vi "timerfd_settime.vi"(8 "error in (no error)":errorcluster, 10 "new value":T1, 11 "fd in":i32) -> (0 "error out":errorcluster, 2 "old value":T1, 3 "fd out":i32)   [LabVIEW 2013, in "Linux RT IPC.C.lvlib"]
uses:
  Linux RT IPC.C.lvlib
  Controls/functions.ctl
  <vilib>/NI/NI Linux RT Errno/Linux Errno.lvlib
  <vilib>/NI/NI Linux RT Utilities/Linux RT Utilities.lvlib
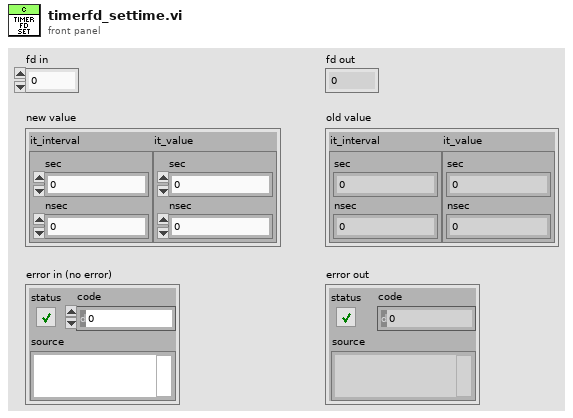
[diagram p1: front panel]
types:
  T1 = cluster{"it_interval":cluster{"sec":u64, "nsec":u64}, "it_value":cluster{"sec":u64, "nsec":u64}}
  T2 = cluster{"it_interval":cluster{"sec":u32, "nsec":u32}, "it_value":cluster{"sec":u32, "nsec":u32}}
  T3 = cluster{"timespec 64":cluster{"sec":u64, "nsec":u64}, "timespec 64":cluster{"sec":u64, "nsec":u64}}
  T4 = typedef "Linux RT IPC.C.lvlib/functions.ctl" = enum16{"unspecified", "close", "epoll_create", "epoll_ctl", "epoll_wait", "fstat", "ftruncate", "mkfifo", "mmap", "munmap", "open", "read", "shm_open", "shm_unlink", "timerfd_create", "timerfd_settime", "timerfd_gettime", "write", "unlink"}
  T5 = typedef "Linux Errno.lvlib/errno.ctl" = enum16{"NO ERROR", "EPERM", "ENOENT", "ESRCH", "EINTR", "EIO", "ENXIO", "E2BIG", "ENOEXEC", "EBADF", "ECHILD", "EAGAIN", "ENOMEM", "EACCES", "EFAULT", "ENOTBLK", "EBUSY", "EEXIST", "EXDEV", "ENODEV", "ENOTDIR", "EISDIR", "EINVAL", "ENFILE", "EMFILE", "ENOTTY", "ETXTBSY", "EFBIG", "ENOSPC", "ESPIPE", "EROFS", "EMLINK", "EPIPE", "EDOM", "ERANGE", "EDADLK", "ENAMETOOLONG", "ENOLCK", "ENOSYS", "ENOTEMPTY", "ELOOP", "EWOULDBLOCK", "ENOMSG", "EIDRM", "ECHRNG", "EL2NSYNC", "EL3HLT", "EL3RST", "ELNRNG", "EUNATCH", "ENOCSI", "EL2HLT", "EBADE", "EBADR", "EXFULL", "ENOANO", "EBADRQC", "EBADSLT", "EDEADLOCK", "EBFONT", "ENOSTR", "ENODATA", "ETIME", "ENOSR", "ENONET", "ENOPKG", "EREMOTE", "ENOLINK", "EADV", "ESRMNT", "ECOMM", "EPROTO", "EMULTIHOP", "EDOTDOT", "EBADMSG", "EOVERFLOW", "ENOTUNIQ", "EBADFD", "EREMCHG", "ELIBACC", "ELIBBAD", "ELIBSCN", "ELIBMAX", "ELIBEXEC", "ELISEQ", "ERESTART", "ESTRPIPE", "EUSERS", "ENOTSOCK", "EDESTADDRREQ", "EMSGSIZE", "EPROTOTYPE", "ENOPROTOOPT", "EPROTONOSUPPORT", "ESOCKTNOSUPPORT", "EOPNOTSUPP", "EPFNOSUPPORT", "EAFNOSUPPORT", "EADDRINUSE", "EADDRNOTAVAIL", "ENETDOWN", "ENETUNREACH", "ENETRESET", "ECONNABORTED", "ECONNRESET", "ENOBUFS", "EISCONN", "ENOTCONN", "ESHUTDOWN", "ETOOMANYREFS", "ETIMEDOUT", "ECONNREFUSED", "EHOSTDOWN", "EHOSTUNREACH", "EALREADY", "EINPROGRESS", "ESTALE", "EUCLEAN", "ENOTNAM", "ENAVAIL", "EISNAM", "EREMOTEIO", "EDQUOT", "ENOMEDIUM", "EMEDIUMTYPE", "ECANCELED", "ENOKEY", "EKEYEXPIRED", "EKEYREVOKED", "EKEYREJECTED", "EOWNERDEAD", "ENOTRECOVERABLE", "ERFKILL", "EHWPOISON", "UNDEFINED"}
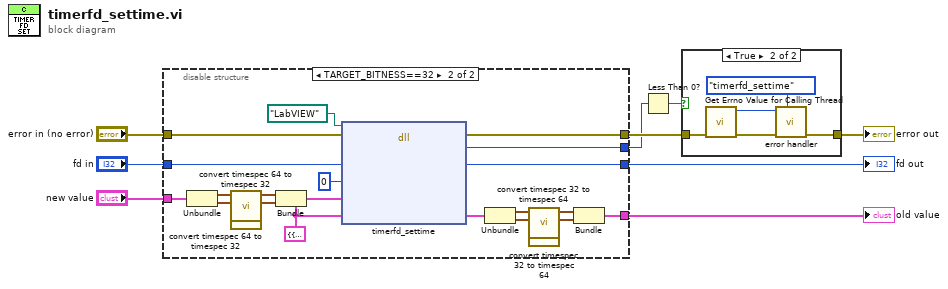
[diagram p0: block diagram]
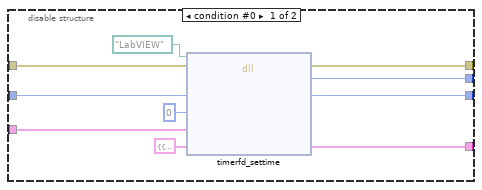
[diagram p2: hidden frame]
diagram:
  n1 = disable-structure shown="TARGET_BITNESS==32" {
    disable-tunnel: "error in (no error)" -> [w19 w39]
    disable-tunnel: [w18 w38] -> w8
    disable-tunnel: "new value" -> [w15 w32]
    disable-tunnel: [w13 w22] -> w4
    disable-tunnel: [w12 w35] -> w1
    disable-tunnel: "fd in" -> [w11 w34]
    disable-tunnel: [w10 w33] -> w2
    frame condition #0 {
      n2 = dll-call lib="LabVIEW" fn="timerfd_settime"(path in=path "LabVIEW", error in=w19, "fd"=w11, "flags"=u16 0, "new_value"=w15, "old_value"=T1 {"it_interval"={"sec"=0, "nsec"=0}, "it_value"={"sec"=0, "nsec"=0}} ("old value")) -> (error out=w18:errorcluster, "return"=w10:i32, "fd"=w12:i32, "old_value"=w13:T1)  [unwired: 3 in, 1 out]
    }
    frame condition #1 (active) {
      w31 = T2 {"it_interval"={"sec"=0, "nsec"=0}, "it_value"={"sec"=0, "nsec"=0}} ("old value")
      n3 = Unbundle(w32) -> ("it_interval"=w29:cluster{"sec":u64, "nsec":u64}, "it_value"=w27:cluster{"sec":u64, "nsec":u64})
      n4 = call <vilib>:"convert timespec 64 to timespec 32.vi"("timespec 64"=w29) -> ("timespec 32"=w28:cluster{"sec":u32, "nsec":u32})  [unwired: 10 in]
      n5 = call <vilib>:"convert timespec 64 to timespec 32.vi"("timespec 64"=w27) -> ("timespec 32"=w26:cluster{"sec":u32, "nsec":u32})  [unwired: 10 in]
      n6 = Bundle(cluster=w31, "it_interval"=w28, "it_value"=w26) -> (w30:T2)
      n7 = dll-call lib="LabVIEW" fn="timerfd_settime"(path in=path "LabVIEW", error in=w39, "fd"=w34, "flags"=u16 0, "new_value"=w30, "old_value"=w31) -> (error out=w38:errorcluster, "return"=w33:i32, "fd"=w35:i32, "old_value"=w23:T2)  [unwired: 3 in, 1 out]
      n8 = Unbundle(w23) -> ("it_interval"=w25:cluster{"sec":u32, "nsec":u32}, "it_value"=w21:cluster{"sec":u32, "nsec":u32})
      n9 = call <vilib>:"convert timespec 32 to timespec 64.vi"("timespec 32"=w25) -> ("timespec 64"=w24:cluster{"sec":u64, "nsec":u64})  [unwired: 10 in]
      n10 = call <vilib>:"convert timespec 32 to timespec 64.vi"("timespec 32"=w21) -> ("timespec 64"=w20:cluster{"sec":u64, "nsec":u64})  [unwired: 10 in]
      n11 = Bundle("timespec 64"=w24, "timespec 64"=w20) -> (w22:T3)  [unwired: 1 in]
    }
  }
  "fd out" <- w1
  "old value" <- w4
  n12 = Less Than 0?(x=w2) -> (x < 0?=w6:bool)
  n13 = case shown="True" w6 {
    tunnel: w8 -> [w40 w45]
    tunnel: [w40 w44] -> w7
    frame False {
    }
    frame True {
      n14 = call <vilib>:"Get Errno Value for Calling Thread.vi"("error in (no error)"=w45) -> ("error out"=w42:errorcluster, "errno"=w43:T5)  [unwired: 9 in]
      n15 = call "error handler.vi"("function (unspecified)"=functions."timerfd_settime" ("function"), "error in (no error)"=w42, "errno"=w43) -> ("error out"=w44:errorcluster)  [unwired: 8 in]
    }
  }
  "error out" <- w7
